vi "To Ref.vi"(10 "error in (no error)":errorcluster, 11 "Config Element in":refnum<class "Config Element.lvclass">) -> (2 "error out":errorcluster)   [LabVIEW 2020]
uses:
  Config Element.lvclass
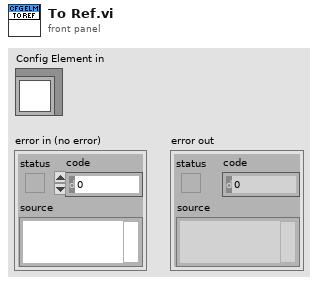
[diagram p1: front panel]
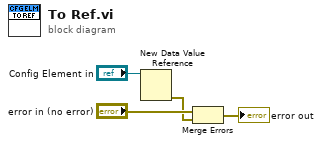
[diagram p0: block diagram]
diagram:
  n1 = New Data Value Reference(data value="Config Element in") -> (data value reference=w1:refnum<data-value>, error out=w2:errorcluster)  [unwired: 1 in]
  n2 = Merge Errors("error in (no error)", w2) -> (→"error out":errorcluster)
